vi "Structure.vi"() -> ()   [LabVIEW 2020]
panel:
  out "Iterateur while":i32
  in  "BTN_Stop":bool
  out "Char_affiche_évènement":string
  in  "BTN_2":bool
  in  "BTN_1":bool
  out "Iterateur":i32
  out "Char_affiche_case":string
  in  "Int_case":u8
  out "Char_affiche_if":string
  in  "BTN_if":bool
  # "IF"
  # "CASE"
  # "For"
  # "Evènement"
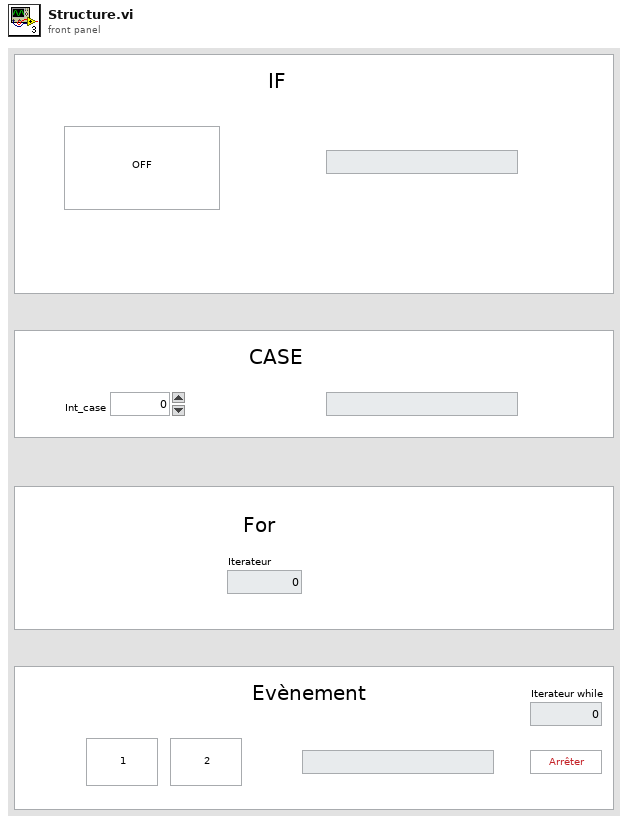
[diagram p1: front panel]
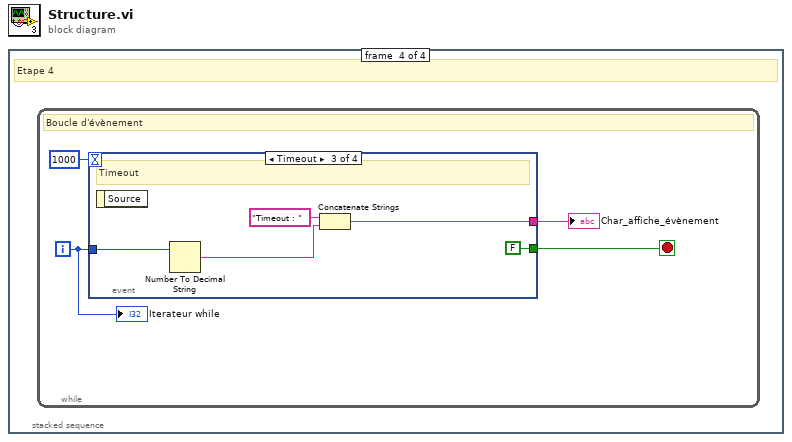
[diagram p0: block diagram]
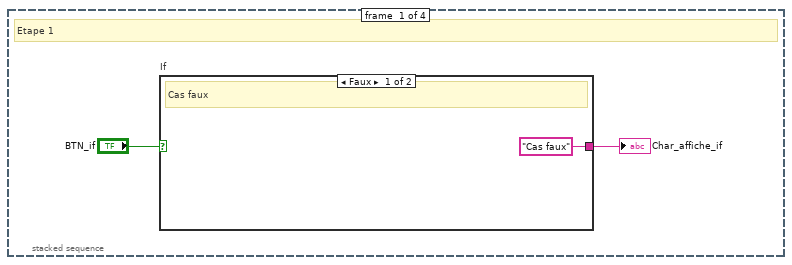
[diagram p2: hidden frame]
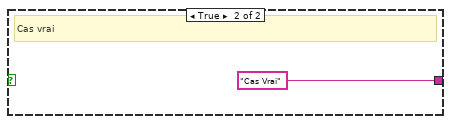
[diagram p3: hidden frame]
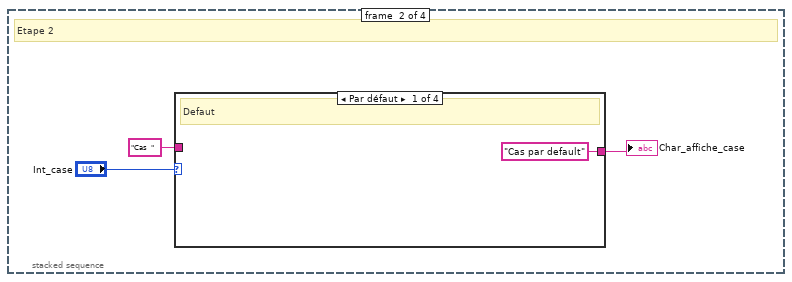
[diagram p4: hidden frame]
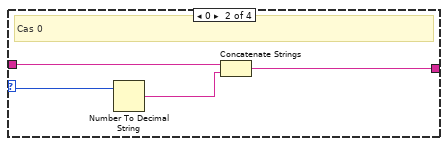
[diagram p5: hidden frame]
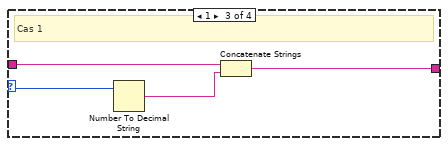
[diagram p6: hidden frame]
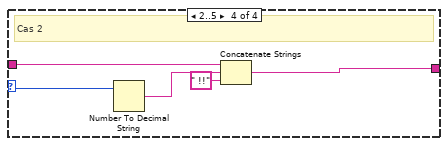
[diagram p7: hidden frame]
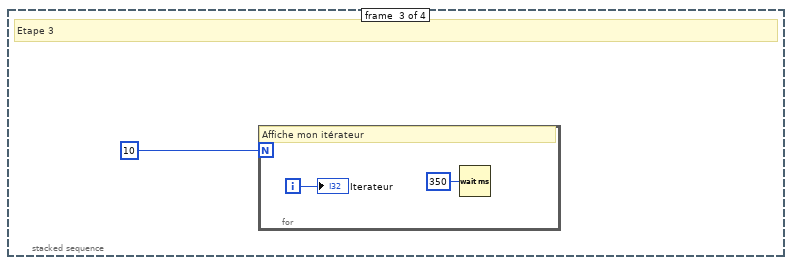
[diagram p8: hidden frame]
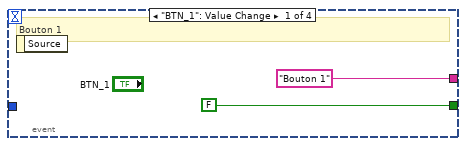
[diagram p9: hidden frame]
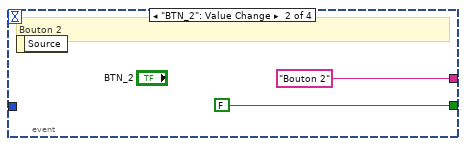
[diagram p10: hidden frame]
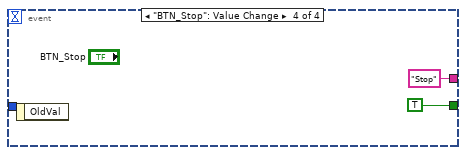
[diagram p11: hidden frame]
diagram:
  n1 = stacked-sequence {
    frame #0 {
      # "Etape 1"
      n2 = case "If" shown="Faux" "BTN_if" {
        tunnel: ["Cas faux" "Cas Vrai"] -> w2
        frame False {
          # "Cas faux"
        }
        frame True {
          # "Cas vrai"
        }
      }
      "Char_affiche_if" <- w2
    }
    frame #1 {
      # "Etape 2"
      n3 = case shown="Par défaut" "Int_case" {
        selector: "Int_case" -> [_ w11 w15 w20]
        tunnel: ["Cas par default" w9 w13 w18] -> w7
        tunnel: "Cas  " -> [_ w12 w16 w21]
        frame Default {
          # "Defaut"
        }
        frame 0 {
          # "Cas 0"
          n4 = Number To Decimal String(number=w11) -> (decimal integer string=w10:string)  [unwired: 1 in]
          n5 = Concatenate Strings(w12, w10) -> (w9:string)
        }
        frame 1 {
          # "Cas 1"
          n6 = Number To Decimal String(number=w15) -> (decimal integer string=w14:string)  [unwired: 1 in]
          n7 = Concatenate Strings(w16, w14) -> (w13:string)
        }
        frame 2..5 {
          # "Cas 2"
          n8 = Number To Decimal String(number=w20) -> (decimal integer string=w19:string)  [unwired: 1 in]
          n9 = Concatenate Strings(w21, w19, " !!" ("chaîne")) -> (w18:string)
        }
      }
      "Char_affiche_case" <- w7
    }
    frame #2 {
      # "Etape 3"
      n10 = for {
        N: 10 -> [_]
        i -> [w24]
        # "Affiche mon itérateur"
        n11 = Wait (ms)(milliseconds to wait=u32 350 ("attente (ms)")) -> ()  [unwired: 1 out]
        "Iterateur" <- w24
      }
    }
    frame #3 {
      # "Etape 4"
      n12 = while {
        i -> [w25]
        stop <- w27 stop-if-true
        # "Boucle d'évènement"
        n13 = event shown="[2] Timeout" {
          selector: _ -> [_ _ _ _]
          dyn-events: _ -> [_ _ _ _]
          timeout: 1000 -> [_ _ _ _]
          tunnel: ["Bouton 1" "Bouton 2" w33 "Stop"] -> w28
          tunnel: [FALSE FALSE FALSE TRUE] -> w27
          tunnel: w25 -> [_ _ w36 _]
          event "BTN_1": Value Change {
            # "Bouton 1"
            n14 = event-data() -> ()  [unwired: 1 in, 1 out]
          }
          event "BTN_2": Value Change {
            # "Bouton 2"
            n15 = event-data() -> ()  [unwired: 1 in, 1 out]
          }
          event Timeout {
            # "Timeout"
            n16 = event-data() -> ()  [unwired: 1 in, 1 out]
            n17 = Number To Decimal String(number=w36) -> (decimal integer string=w35:string)  [unwired: 1 in]
            n18 = Concatenate Strings("Timeout : " ("chaîne"), w35) -> (w33:string)
          }
          event "BTN_Stop": Value Change {
            n19 = event-data() -> ()  [unwired: 1 in, 1 out]
          }
        }
        "Char_affiche_évènement" <- w28
        "Iterateur while" <- w25
      }
    }
  }
